vi "Decode_UICTextFiles.vi"(8 "error in":errorcluster, 10 "Text Array":string[](array[string])) -> (0 "error out":errorcluster, 1 "Spectrum":T1={"SampleRate"=-1.0, "TrigDelay"=0.0, "SpecLength"=0.0, "DAQ_Range"=0.0, "Average#"=0, "Position"=[], "Spectrum"=[], "Calibr."=[], "Pressure"=-1.0, "Desp_LaserEnergy"=-1.0, "PI_LaserEnergy"=-1.0, "Voltages Table"=[], "ProcMode"=enum."None", "Threshold"=-1.0, "Comment"="", "TickCount"=0.0, "Time Stamp"=timestamp(0 s since 1904-01-01)} {"TickCount" format="%#.2f"}, 2 "Signal":dbl[](array[numeric]), 3 "m/z list":dbl[](array[numeric]), 4 "InitialCali.":dbl[](array[numeric]))   [LabVIEW 2013]
uses:
  Files/Signal_Segment.ctl
  ControlDef/ProcessingMode.ctl
panel:
  out "Headerlines":string[](array[string])
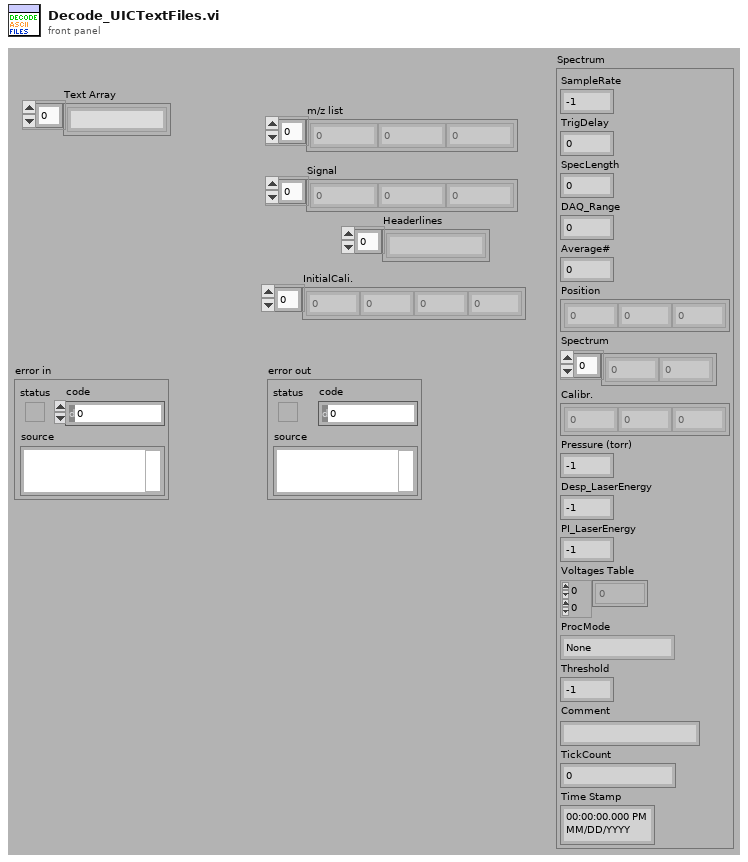
[diagram p1: front panel]
types:
  T1 = typedef "Signal_Segment.ctl" = cluster{"SampleRate":dbl, "TrigDelay":dbl, "SpecLength":dbl, "DAQ_Range":dbl, "Average#":i32, "Position":dbl[], "Spectrum":sgl[], "Calibr.":dbl[], "Pressure":dbl, "Desp_LaserEnergy":dbl, "PI_LaserEnergy":dbl, "Voltages Table":sgl[][], "ProcMode":T2, "Threshold":dbl, "Comment":string, "TickCount":dbl, "Time Stamp":timestamp}
  T2 = typedef "ProcessingMode.ctl" = enum16{"None", "Drop by Threshold", "TDC Simulate", "SetFilter"}
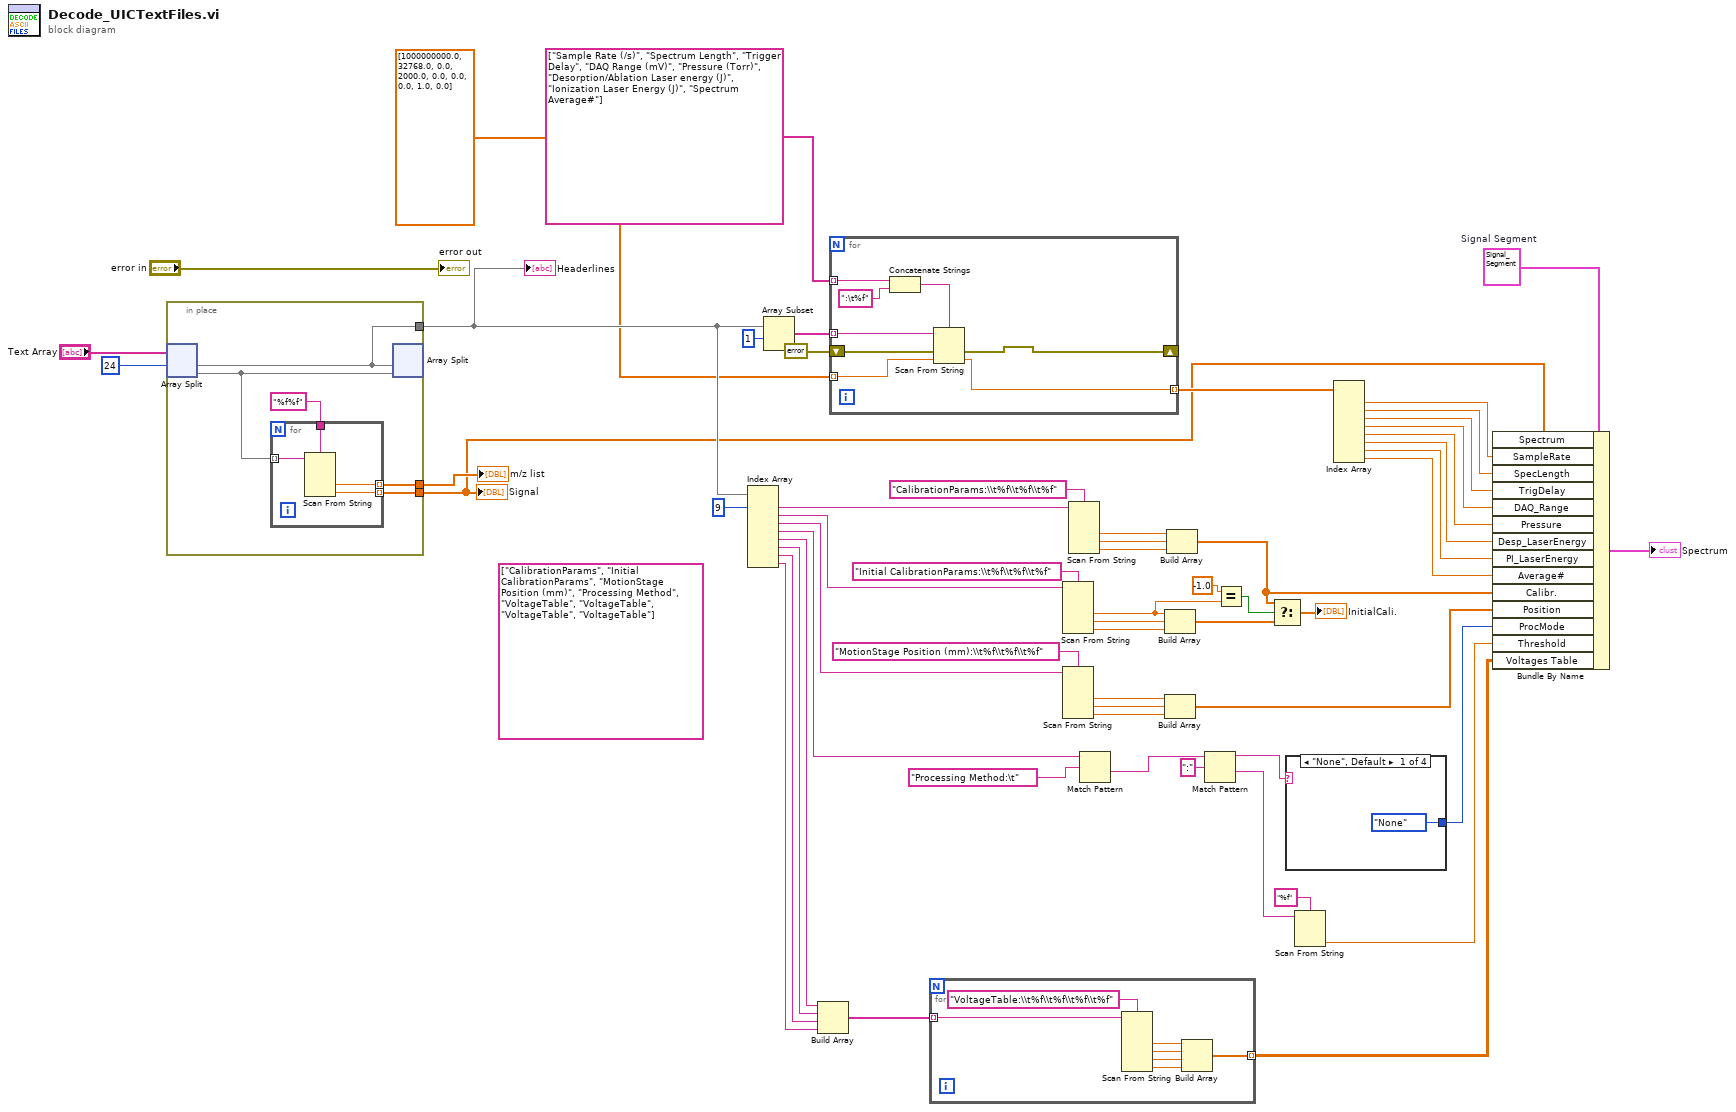
[diagram p0: block diagram]
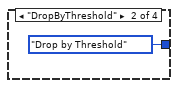
[diagram p2: hidden frame]
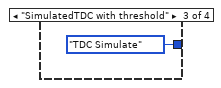
[diagram p3: hidden frame]
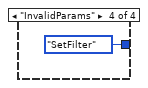
[diagram p4: hidden frame]
diagram:
  (unwired) string[] ["CalibrationParams", "Initial CalibrationParams", "MotionStage Position (mm)", "Processing Method", "VoltageTable", "VoltageTable", "VoltageTable", "VoltageTable"]
  w55 = T1 {"SampleRate"=-1.0, "TrigDelay"=0.0, "SpecLength"=0.0, "DAQ_Range"=0.0, "Average#"=0, "Position"=[], "Spectrum"=[], "Calibr."=[], "Pressure"=-1.0, "Desp_LaserEnergy"=-1.0, "PI_LaserEnergy"=-1.0, "Voltages Table"=[], "ProcMode"=enum."None", "Threshold"=-1.0, "Comment"="", "TickCount"=0.0, "Time Stamp"=timestamp(0 s since 1904-01-01)}  # Signal Segment
  n1 = in-place {
    in-place-border: [w62] -> w56
    in-place-border: [w61] -> w8
    in-place-border: [w60] -> w51
    n2 = in-place-split #1("Text Array", 24 ("index")) -> (w60:string[], w63:string[])
    n3 = for {
      tunnel: [w65] -> w61 mode=indexing
      tunnel: "%f%f" ("format string") -> [w68]
      tunnel: w63 -> [w67] mode=indexing
      tunnel: [w66] -> w62 mode=indexing
      n4 = Scan From String(format string=w68, input string=w67) -> (output 1=w66:dbl, output 2=w65:dbl)  [unwired: 4 in, 3 out]
    }
    n5 = in-place-split #1(w60, w63) -> ()  [unwired: 2 out]
  }
  "Signal" <- w8
  "m/z list" <- w56
  "Headerlines" <- w51
  n6 = Index Array(array=w51, index #1=9 ("length")) -> (element #1=w49:string, element #2=w46:string, element #3=w44:string, element #4=w19:string, element #5=w35:string, element #6=w34:string, element #7=w33:string, element #8=w32:string)  [unwired: 7 in]
  n7 = Array Subset(array=w51, index=1) -> (w54:string[])  [unwired: 1 in]
  n8 = Build Array(w35, w34, w33, w32) -> (w31:string[])
  n9 = for {
    tunnel: w54 -> [w76] mode=indexing
    shift-right: [w75] -> _
    shift-left: errorcluster {"status"=FALSE, "code"=0, "source"=""} ("error IO") -> [w74]
    tunnel: string[] ["Sample Rate (/s)", "Spectrum Length", "Trigger Delay", "DAQ Range (mV)", "Pressure (Torr)", "Desorption/Ablation Laser energy (J)", "Ionization Laser Energy (J)", "Spectrum Average#"] -> [w73] mode=indexing
    tunnel: [w70] -> w28 mode=indexing
    tunnel: dbl[] [1000000000.0, 32768.0, 0.0, 2000.0, 0.0, 0.0, 0.0, 1.0, 0.0] -> [w69] mode=indexing
    n10 = Concatenate Strings(w73, ":\t%f" ("format string")) -> (w71:string)
    n11 = Scan From String(format string=w71, input string=w76, error in=w74, default 1=w69) -> (error out=w75:errorcluster, output 1=w70:dbl)  [unwired: 1 in, 2 out]
  }
  n12 = for {
    tunnel: w31 -> [w82] mode=indexing
    tunnel: [w77] -> w10 mode=indexing
    n13 = Scan From String(format string="VoltageTable:\\t%f\\t%f\\t%f\\t%f", input string=w82) -> (output 1=w81:dbl, output 2=w80:dbl, output 3=w79:dbl, output 4=w78:dbl)  [unwired: 6 in, 3 out]
    n14 = Build Array(w81, w80, w79, w78) -> (w77:dbl[])
  }
  n15 = Scan From String(format string="Initial CalibrationParams:\\t%f\\t%f\\t%f", input string=w46) -> (output 1=w5:dbl, output 2=w39:dbl, output 3=w40:dbl)  [unwired: 5 in, 3 out]
  n16 = Scan From String(format string="MotionStage Position (mm):\\t%f\\t%f\\t%f", input string=w44) -> (output 1=w43:dbl, output 2=w42:dbl, output 3=w41:dbl)  [unwired: 5 in, 3 out]
  n17 = Scan From String(format string="CalibrationParams:\\t%f\\t%f\\t%f", input string=w49) -> (output 1=w36:dbl, output 2=w37:dbl, output 3=w38:dbl)  [unwired: 5 in, 3 out]
  n18 = Match Pattern(string=w19, regular expression="Processing Method:\t" ("format string")) -> (after substring=w17:string)  [unwired: 1 in, 3 out]
  n19 = Build Array(w5, w39, w40) -> (w2:dbl[])
  n20 = Build Array(w43, w42, w41) -> (w30:dbl[])
  n21 = Build Array(w36, w37, w38) -> (w3:dbl[])
  n22 = Match Pattern(string=w17, regular expression=":") -> (before substring=w12:string, after substring=w15:string)  [unwired: 1 in, 2 out]
  n23 = Equal?(x=-1.0 ("y"), y=w5) -> (x = y?=w6:bool)
  n24 = Select(t=w3, s=w6, f=w2) -> (s? t:f=→"InitialCali.":dbl[])
  n25 = case shown="\"None\", Default" w12 {
    tunnel: [ProcessingMode."None" ("ProcMode") ProcessingMode."Drop by Threshold" ("ProcMode") ProcessingMode."TDC Simulate" ("ProcMode") ProcessingMode."SetFilter" ("ProcMode")] -> w11
    frame "None", Default {
    }
    frame "DropByThreshold" {
    }
    frame "SimulatedTDC with threshold" {
    }
    frame "InvalidParams" {
    }
  }
  n26 = Scan From String(format string="%f", input string=w15) -> (output 1=w13:dbl)  [unwired: 3 in, 3 out]
  n27 = Index Array(array=w28) -> (element #1=w27:dbl, element #2=w26:dbl, element #3=w25:dbl, element #4=w24:dbl, element #5=w23:dbl, element #6=w22:dbl, element #7=w21:dbl, element #8=w20:dbl)  [unwired: 8 in]
  n28 = Bundle By Name(cluster=w55, "Spectrum"=w8, "SampleRate"=w27, "SpecLength"=w26, "TrigDelay"=w25, "DAQ_Range"=w24, "Pressure"=w23, "Desp_LaserEnergy"=w22, "PI_LaserEnergy"=w21, "Average#"=w20, "Calibr."=w3, "Position"=w30, "ProcMode"=w11, "Threshold"=w13, "Voltages Table"=w10) -> (→"Spectrum":T1)
  "error out" <- "error in"
